vi "TCP Parse Address-Port.vi"(0 "TCP address:port":string="192.168.0.3:502") -> (1 "port":u16, 2 "address":string)   [LabVIEW 2010]
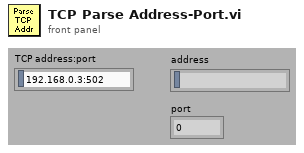
[diagram p1: front panel]
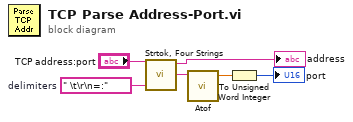
[diagram p0: block diagram]
diagram:
  w6 = " \t\r\n=:"  # delimiters
  n1 = call "Strtok, Four Strings.vi"("delimiters (\\s\\t\\r\\n=)"=w6, "input string"="TCP address:port") -> ("token 2"=w4:string, "token 1"=→"address":string)  [unwired: 1 in, 2 out]
  n2 = call "Atof.vi"("string"=w4) -> ("number"=w5:dbl)  [unwired: 6 in]
  n3 = To Unsigned Word Integer(number=w5) -> (unsigned 16bit integer=→"port":u16)
